vi "write syslog.vi"(6 "prog":string, 7 "Facility":T1(ring)=enum."user", 8 "error in (no error)":errorcluster, 9 "Minimum level to log":T2(ring)=enum."Debug", 10 "Priority":T2(ring)=enum."Debug", 11 "msg":string) -> (0 "error out":errorcluster)   [LabVIEW 2013]
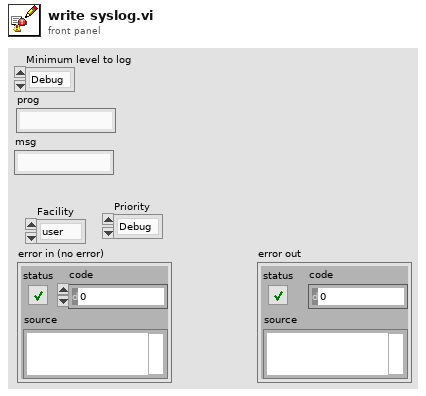
[diagram p1: front panel]
types:
  T1 = enum16{"kern", "user", "mail", "daemon", "auth", "syslog", "lpr", "news", "uucp", "clk", "authpriv", "ftp", "NTP", "log audit", "log alert", "cron", "local0", "local1", "local2", "local3", "local4", "local5", "local6", "local7"}
  T2 = enum16{"Emergency", "Alert", "Critical", "Error", "Warning", "Notice", "Informational", "Debug"}
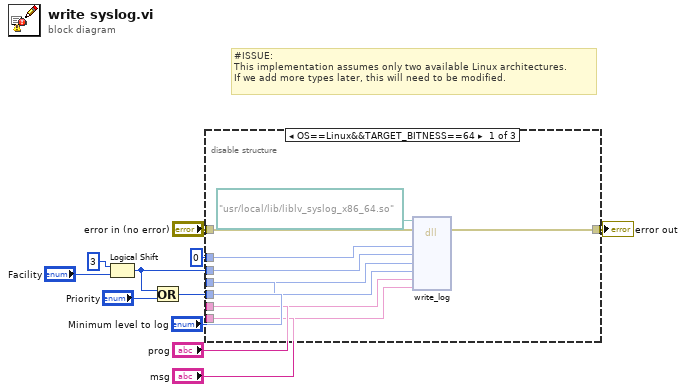
[diagram p0: block diagram]
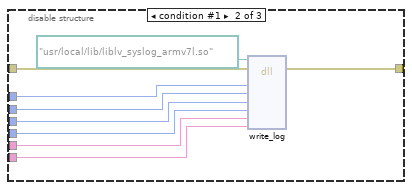
[diagram p2: hidden frame]
diagram:
  # "#ISSUE:\nThis implementation assumes only two available Linux architectures.\nIf we add more types later, this will need to be modified."
  n1 = Logical Shift(y=i16 3 ("n"), x="Facility") -> (x << y=w4:u32)
  n2 = Or(x=w4, y="Priority") -> (x .or. y?=w3:u32)
  n3 = disable-structure shown="OS==Linux&&TARGET_BITNESS==64" {
    disable-tunnel: "Minimum level to log" -> [w20 w29 _]
    disable-tunnel: "prog" -> [w19 w28 _]
    disable-tunnel: "msg" -> [w18 w27 _]
    disable-tunnel: 0 -> [w17 w26 _]
    disable-tunnel: [w16 w25 w30] -> w7
    disable-tunnel: w4 -> [w15 w24 _]
    disable-tunnel: w3 -> [w14 w23 _]
    disable-tunnel: "error in (no error)" -> [w13 w22 w30]
    frame condition #0 {
      n4 = dll-call lib="C:/Users/MatthewPollock/Documents/GitHub/syslog/source/liblv_syslog_x86_64.*" fn="write_log"(path in=path "/usr/local/lib/liblv_syslog_x86_64.so", error in=w13, "option"=w17, "facility"=w15, "priority"=w14, "mask"=w20, "prog"=w19, "msg"=w18) -> (error out=w16:errorcluster)  [unwired: 8 in, 1 out]
    }
    frame condition #1 {
      n5 = dll-call lib="C:/Users/MatthewPollock/Documents/GitHub/syslog/source/liblv_syslog_armv7l.*" fn="write_log"(path in=path "/usr/local/lib/liblv_syslog_armv7l.so", error in=w22, "option"=w26, "facility"=w24, "priority"=w23, "mask"=w29, "prog"=w28, "msg"=w27) -> (error out=w25:errorcluster)  [unwired: 8 in, 1 out]
    }
    frame condition #2 (active) {
      # "#TODO:\nThrow unsupported OS error"
    }
  }
  "error out" <- w7
